vi "Test_salEvent_logLevel.vi"(8 "error in (no error)":errorcluster) -> (0 "error out":errorcluster, 3 "function return":i32)   [LabVIEW 2018, in "SALLV_Test.lvlib"]
doc: "int Test_shm_salEvent_logLevelLV();"
uses:
  SALLV_Test.lvlib
  SALLV_Test.so
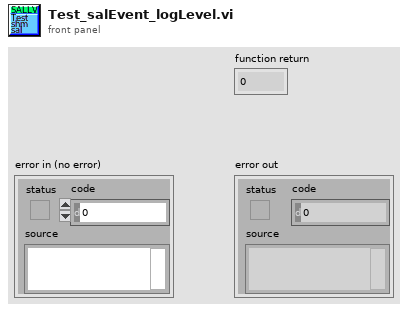
[diagram p1: front panel]
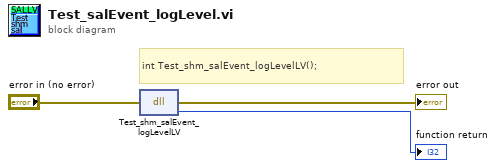
[diagram p0: block diagram]
diagram:
  # "int Test_shm_salEvent_logLevelLV();"
  n1 = dll-call lib="home/ttsai/Documents/github/ts_SALLabVIEW/testPerfTemp/TestData/SALLV_Test.*" fn="Test_shm_salEvent_logLevelLV"(error in="error in (no error)") -> (error out=→"error out":errorcluster, →"function return":i32)  [unwired: 2 in, 1 out]
